vi "Unit Test - Replace CSM - Internal State Debug Log History.vi"() -> (0 "error out":errorcluster)   [LabVIEW 2017, in "testcase-csmhelper.lvclass"]
uses:
  testcase-csmhelper.lvclass
  src/user.lib/_NEVSTOP/Communicable State Machine(CSM)/_csmHelper/API/Create From VI Reference.vi
  src/user.lib/_NEVSTOP/Communicable State Machine(CSM)/_csmHelper/API/Start Undo.vi
  src/user.lib/_NEVSTOP/Communicable State Machine(CSM)/_csmHelper/usecase/Replace Debug Log History Method.vi
  src/user.lib/_NEVSTOP/Communicable State Machine(CSM)/_csmHelper/API/Stop Undo.vi
  src/user.lib/_NEVSTOP/Communicable State Machine(CSM)/_csmHelper/API/Undo.vi
  src/user.lib/_NEVSTOP/Communicable State Machine(CSM)/_csmHelper/API/Destroy.vi
  src/user.lib/_NEVSTOP/Communicable State Machine(CSM)/_csmHelper/CSM-Helper.lvclass
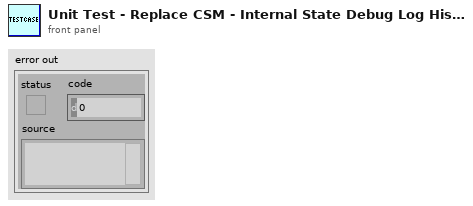
[diagram p1: front panel]
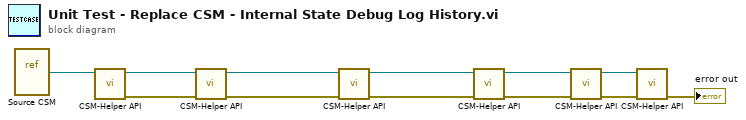
[diagram p0: block diagram]
diagram:
  n1 = vi-ref "Source CSM.vi"() -> (w12:refnum<vi>)
  n2 = call-poly "CSM-Helper API.vi"("VI"=w12) -> ("error out"=w10:errorcluster, "CSM-Helper.lvclass"=w9:refnum<class "CSM-Helper.lvclass">)  [unwired: 9 in]
  n3 = call-poly "CSM-Helper API.vi"("error in (no error)"=w10, "CSM-Helper in"=w9) -> ("error out"=w8:errorcluster, "CSM-Helper out"=w7:refnum<class "CSM-Helper.lvclass">)  [unwired: 8 in]
  n4 = call-poly "CSM-Helper API.vi"("error in (no error)"=w8, "CSM-Helper in"=w7) -> ("error out"=w1:errorcluster, "CSM-Helper out"=w2:refnum<class "CSM-Helper.lvclass">)  [unwired: 8 in]
  n5 = call-poly "CSM-Helper API.vi"("error in (no error)"=w1, "CSM-Helper in"=w2) -> ("error out"=w6:errorcluster, "CSM-Helper out"=w5:refnum<class "CSM-Helper.lvclass">)  [unwired: 8 in]
  n6 = call-poly "CSM-Helper API.vi"("error in (no error)"=w6, "CSM-Helper in"=w5) -> ("error out"=w4:errorcluster, "CSM-Helper out"=w3:refnum<class "CSM-Helper.lvclass">)  [unwired: 8 in]
  n7 = call-poly "CSM-Helper API.vi"("error in (no error)"=w4, "CSM-Helper in"=w3) -> ("error out"=→"error out":errorcluster)  [unwired: 8 in, 1 out]
